vi "SetAutoShutter.vi"(8 "error in (no error)":errorcluster, 9 "Value":bool=TRUE, 10 "Label":string, 11 "Laser_Oxxius in":refnum<class "Laser_Oxxius.lvclass">) -> (0 "error out":errorcluster, 3 "Laser_Oxxius out":refnum<class "Laser_Oxxius.lvclass">)   [LabVIEW 2020, in "Laser_Oxxius.lvlib" / "Laser_Oxxius.lvclass"]
uses:
  Laser_Oxxius.lvclass
  Laser_Oxxius.lvclass/Laser_Oxxius.ctl
  D:/Daguan/Development/MMicroscopyAF/Model/Hardware Layer/Real Hardware/Laser_Oxxius/Laser_Oxxius/Dependency/Oxxius_Boxx.dll
  Dependency/Oxxius_Boxx.dll
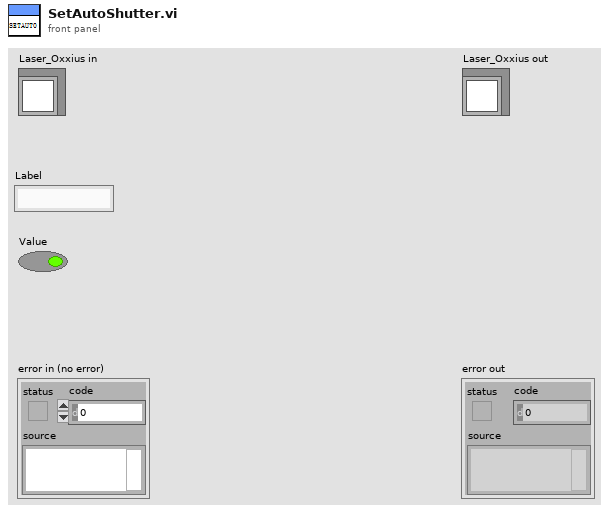
[diagram p1: front panel]
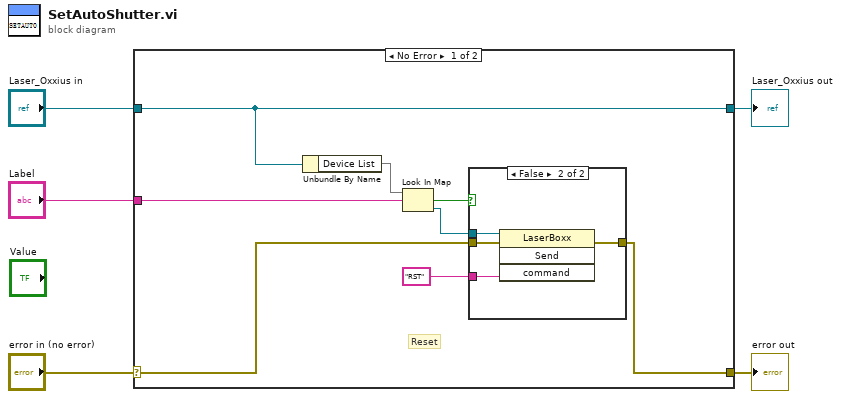
[diagram p0: block diagram]
diagram:
  n1 = case shown="No Error" "error in (no error)" {
    selector: "error in (no error)" -> [w8 w20]
    tunnel: [w7 w20] -> w4
    tunnel: [w10 w19] -> w2
    tunnel: "Laser_Oxxius in" -> [w10 w19]
    tunnel: "Label" -> [w9 _]
    frame No Error {
      # "Reset"
      n2 = Unbundle By Name(w10) -> ("Device List"=w13:map{string, refnum<k24>})
      n3 = Look In Map(map=w13, key=w9) -> (key not found?=w11:bool, value=w12:refnum<k24>)  [unwired: 1 in]
      n4 = case shown="False" w11 {
        tunnel: w8 -> [w14 w18]
        tunnel: w12 -> [_ w17]
        tunnel: [w14 w16] -> w7
        tunnel: "RST" ("command") -> [_ w15]
        frame True {
        }
        frame False {
          n5 = invoke class="LaserBoxx" method="Send"(reference=w17, error in=w18, "command"=w15) -> (error out=w16:errorcluster)  [unwired: 1 in, 3 out]
        }
      }
    }
    frame Error {
    }
  }
  "error out" <- w4
  "Laser_Oxxius out" <- w2
